vi "Run Command Gavin.vi"(2 "Line Index In":i32, 3 "Script":string) -> (0 "Line Index Out":i32, 1 "Done":bool)   [LabVIEW 2017, in "Apple script.lvlib"]
doc: "Looks at a line and runs the appropriate command. Add new commands to this vi."
uses:
  Apple script.lvlib
  Robot Global Data.vi
  <vilib>/addons/control/pid/pid.llb/PID.vi
  <vilib>/addons/control/pid/pid.llb/PID (DBL).vi
  Support Code/Angle Distance.vi
  Support Code/Pigeon Gyro.vi
  Support Code/Encoders.vi
  <vilib>/Rock Robotics/Network Tables/NT Write Value.vi
  <vilib>/Rock Robotics/Network Tables/NT Write Numeric Array.vi
  Parse Number.vi
  Timer.vi
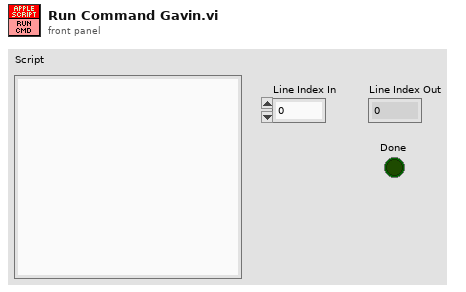
[diagram p1: front panel]
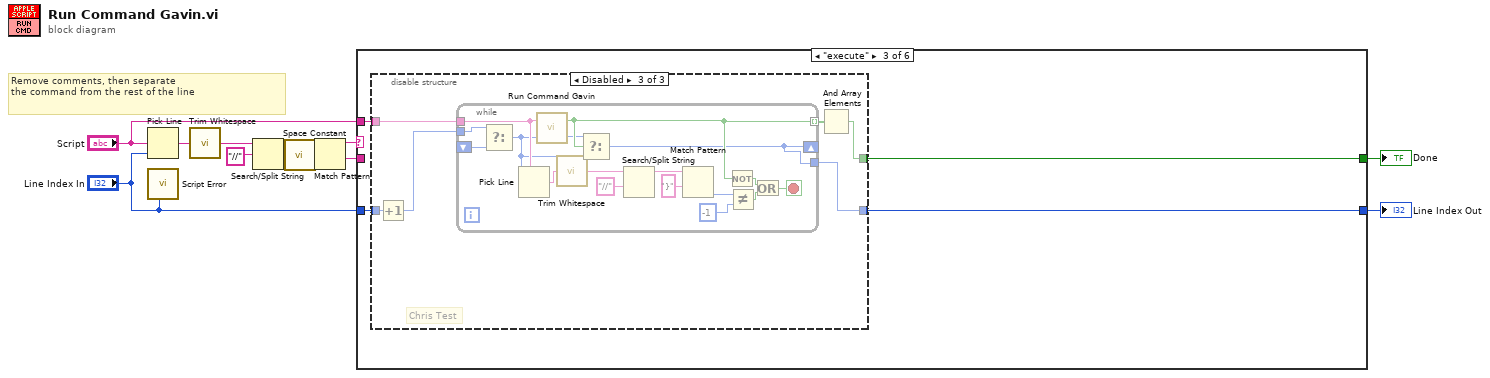
[diagram p0: block diagram]
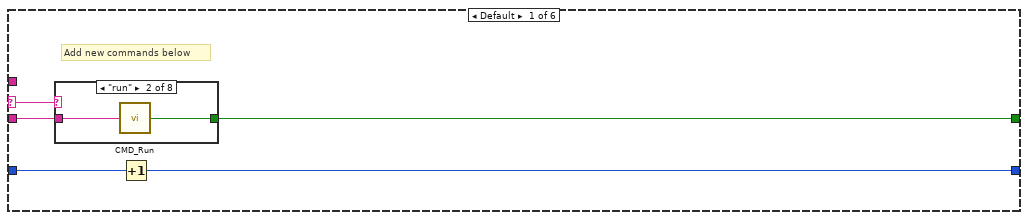
[diagram p2: hidden frame]
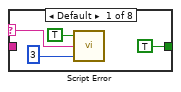
[diagram p3: hidden frame]
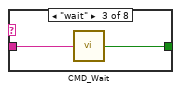
[diagram p4: hidden frame]
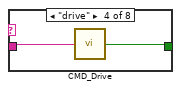
[diagram p5: hidden frame]
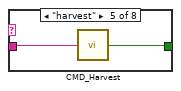
[diagram p6: hidden frame]
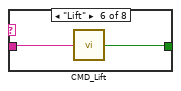
[diagram p7: hidden frame]
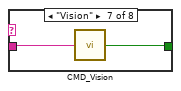
[diagram p8: hidden frame]
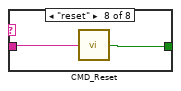
[diagram p9: hidden frame]
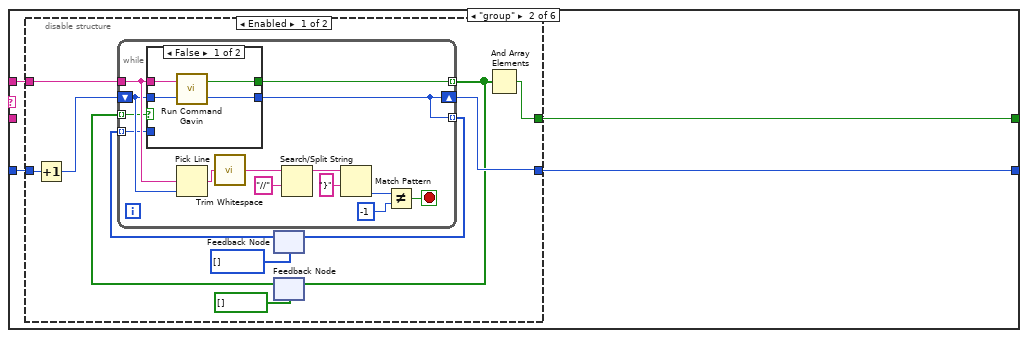
[diagram p10: hidden frame]
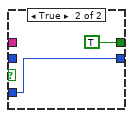
[diagram p11: hidden frame]
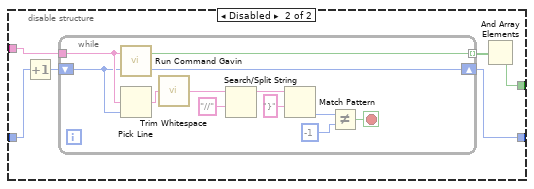
[diagram p12: hidden frame]
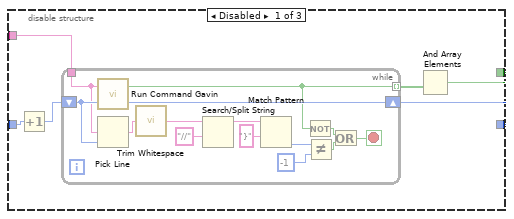
[diagram p13: hidden frame]
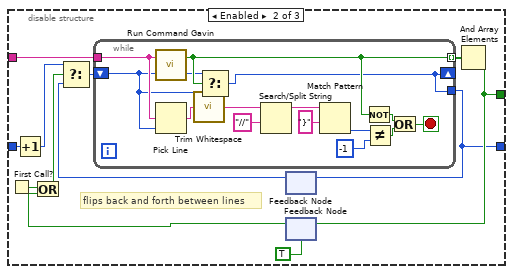
[diagram p14: hidden frame]
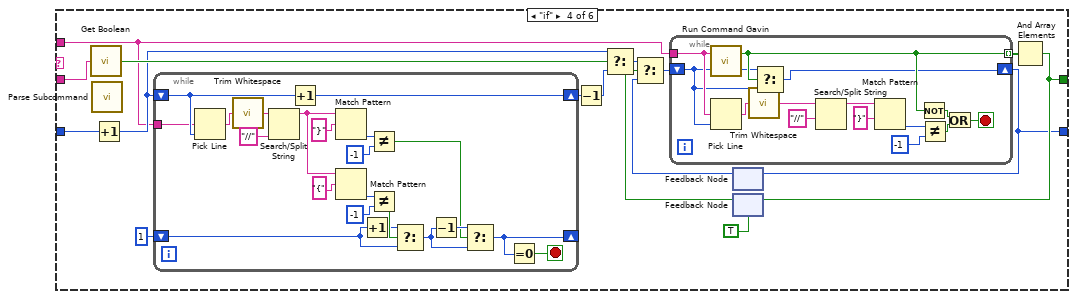
[diagram p15: hidden frame]
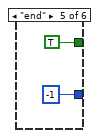
[diagram p16: hidden frame]
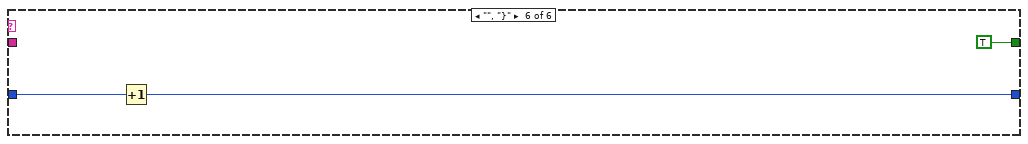
[diagram p17: hidden frame]
diagram:
  # "Remove comments, then separate\nthe command from the rest of the line"
  n1 = Pick Line(multi-line string="Script", line index="Line Index In") -> (output string=w8:string)  [unwired: 1 in]
  n2 = call "Script Error.vi"("Line Number"="Line Index In") -> ()  [unwired: 4 in, 1 out]
  n3 = call <vilib>:"Trim Whitespace.vi"("string"=w8) -> ("trimmed string"=w6:string)  [unwired: 1 in]
  n4 = Search/Split String(string=w6, search string/char (-)="//") -> (substring before match=w5:string)  [unwired: 1 in, 2 out]
  n5 = call <vilib>:"Space Constant.vi"() -> ("String"=w11:string)
  n6 = Match Pattern(string=w5, regular expression=w11) -> (before substring=w4:string, after substring=w3:string)  [unwired: 1 in, 2 out]
  n7 = case shown="\"execute\"" w4 {
    selector: w4 -> [w14 _ _ _ _ _]
    tunnel: "Script" -> [_ w38 w88 w164 _ _]
    tunnel: "Line Index In" -> [w16 w36 w89 w176 _ w217]
    tunnel: [w13 w35 w91 w177 TRUE ("Running") TRUE ("Running")] -> w2
    tunnel: [w15 w37 w90 w174 -1 ("Line Index Out") w216] -> w1
    tunnel: w3 -> [w12 _ _ w175 _ _]
    frame Default {
      # "Add new commands below"
      n8 = case shown="\"run\"" w14 {
        selector: w14 -> [w17 _ _ _ _ _ _ _]
        tunnel: [TRUE w21 w24 w25 w27 w29 w31 w33] -> w13
        tunnel: w12 -> [_ w22 w23 w26 w28 w30 w32 w34]
        frame Default {
          n9 = call "Script Error.vi"("Error?"=TRUE, "Error Details"=w17, "Error Code"=3) -> ()  [unwired: 2 in, 1 out]
        }
        frame "run" {
          n10 = call "CMD_Run.vi"("Line"=w22) -> ("Done"=w21:bool)
        }
        frame "wait" {
          n11 = call "CMD_Wait.vi"("Line"=w23) -> ("Done"=w24:bool)
        }
        frame "drive" {
          n12 = call "CMD_Drive.vi"("Line"=w26) -> ("Done"=w25:bool)
        }
        frame "harvest" {
          n13 = call "CMD_Harvest.vi"("Line"=w28) -> ("Done"=w27:bool)
        }
        frame "Lift" {
          n14 = call "CMD_Lift.vi"("Line"=w30) -> ("Done"=w29:bool)
        }
        frame "Vision" {
          n15 = call "CMD_Vision.vi"("Line"=w32) -> ("Done"=w31:bool)
        }
        frame "reset" {
          n16 = call "CMD_Reset.vi"("Line"=w34) -> ("Done"=w33:bool)
        }
      }
      n17 = Increment(x=w16) -> (x+1=w15:i32)
    }
    frame "group" {
      n18 = disable-structure shown="Enabled" {
        disable-tunnel: w38 -> [w47 w75]
        disable-tunnel: [w48 w72] -> w37
        disable-tunnel: w36 -> [w46 w74]
        disable-tunnel: [w49 w70] -> w35
        frame Enabled {
          n19 = Increment(x=w46) -> (x+1=w42:i32)
          n20 = feedback #1(i32[] []) -> (w41:i32[])
          n21 = feedback #2(bool[] []) -> (w44:bool[])
          n22 = while {
            tunnel: w47 -> [w63]
            tunnel: [w56] -> w45 mode=indexing
            shift-right: [w51] -> w48
            shift-left: w42 -> [w55]
            tunnel: w44 -> [w52] mode=indexing
            tunnel: [w51] -> w43 mode=indexing
            tunnel: w41 -> [w50] mode=indexing
            stop <- w53 stop-if-true
            n23 = case shown="False" w52 {
              tunnel: w63 -> [w67 _]
              tunnel: [w66 TRUE ("Done")] -> w56
              tunnel: w55 -> [w65 _]
              tunnel: [w64 w68] -> w51
              tunnel: w50 -> [_ w68]
              frame False {
                n24 = call "Run Command Gavin.vi"("Line Index In"=w65, "Script"=w67) -> ("Line Index Out"=w64:i32, "Done"=w66:bool)
              }
              frame True {
              }
            }
            n25 = Pick Line(multi-line string=w63, line index=w55) -> (output string=w58:string)  [unwired: 1 in]
            n26 = call <vilib>:"Trim Whitespace.vi"("string"=w58) -> ("trimmed string"=w59:string)  [unwired: 1 in]
            n27 = Search/Split String(string=w59, search string/char (-)="//") -> (substring before match=w54:string)  [unwired: 1 in, 2 out]
            n28 = Match Pattern(string=w54, regular expression="}" ("search string/char (-)")) -> (offset past match=w61:i32)  [unwired: 1 in, 3 out]
            n29 = Not Equal?(x=w61, y=-1) -> (x != y?=w53:bool)
          }
          n30 = feedback-in #1(w43) -> ()
          n31 = feedback-in #2(w45) -> ()
          n32 = And Array Elements(Boolean array=w45) -> (logical AND=w49:bool)
        }
        frame Disabled {
          n33 = Increment(x=w74) -> (x+1=w73:i32)
          n34 = while {
            tunnel: w75 -> [w87]
            tunnel: [w80] -> w71 mode=indexing
            shift-right: [w77] -> w72
            shift-left: w73 -> [w79]
            stop <- w78 stop-if-true
            n35 = call "Run Command Gavin.vi"("Line Index In"=w79, "Script"=w87) -> ("Line Index Out"=w77:i32, "Done"=w80:bool)
            n36 = Pick Line(multi-line string=w87, line index=w79) -> (output string=w82:string)  [unwired: 1 in]
            n37 = call <vilib>:"Trim Whitespace.vi"("string"=w82) -> ("trimmed string"=w83:string)  [unwired: 1 in]
            n38 = Search/Split String(string=w83, search string/char (-)="//") -> (substring before match=w76:string)  [unwired: 1 in, 2 out]
            n39 = Match Pattern(string=w76, regular expression="}" ("search string/char (-)")) -> (offset past match=w85:i32)  [unwired: 1 in, 3 out]
            n40 = Not Equal?(x=w85, y=-1) -> (x != y?=w78:bool)
          }
          n41 = And Array Elements(Boolean array=w71) -> (logical AND=w70:bool)
        }
      }
    }
    frame "execute" {
      n42 = disable-structure shown="Disabled" {
        disable-tunnel: [w94 w116 w141] -> w91
        disable-tunnel: [w95 w112 w139] -> w90
        disable-tunnel: w89 -> [w93 w123 w144]
        disable-tunnel: w88 -> [w96 w121 w142]
        frame Disabled {
          n43 = Increment(x=w93) -> (x+1=w92:i32)
          n44 = while {
            tunnel: w96 -> [w103]
            tunnel: [w99] -> w97 mode=indexing
            shift-right: [w111] -> w95
            shift-left: w92 -> [w104]
            stop <- w102 stop-if-true
            n45 = call "Run Command Gavin.vi"("Line Index In"=w104, "Script"=w103) -> ("Line Index Out"=w111:i32, "Done"=w99:bool)
            n46 = Pick Line(multi-line string=w103, line index=w104) -> (output string=w106:string)  [unwired: 1 in]
            n47 = call <vilib>:"Trim Whitespace.vi"("string"=w106) -> ("trimmed string"=w107:string)  [unwired: 1 in]
            n48 = Search/Split String(string=w107, search string/char (-)="//") -> (substring before match=w98:string)  [unwired: 1 in, 2 out]
            n49 = Match Pattern(string=w98, regular expression="}" ("search string/char (-)")) -> (offset past match=w109:i32)  [unwired: 1 in, 3 out]
            n50 = Not(x=w99) -> (.not. x?=w100:bool)
            n51 = Not Equal?(x=w109, y=-1) -> (x != y?=w101:bool)
            n52 = Or(x=w100, y=w101) -> (x .or. y?=w102:bool)
          }
          n53 = And Array Elements(Boolean array=w97) -> (logical AND=w94:bool)
        }
        frame Enabled {
          # "flips back and forth between lines"
          n54 = First Call?() -> (First Call?: T/F=w113:bool)
          n55 = Increment(x=w123) -> (x+1=w119:i32)
          n56 = feedback #3() -> (w118:i32)  [unwired: 1 in]
          n57 = feedback #4(TRUE) -> (w117:bool)
          n58 = Or(x=w113, y=w117) -> (x .or. y?=w114:bool)
          n59 = Select(t=w119, s=w114, f=w118) -> (s? t:f=w120:i32)
          n60 = while {
            tunnel: w121 -> [w138]
            tunnel: [w128] -> w122 mode=indexing
            shift-right: [w124] -> _
            shift-left: w120 -> [w126]
            tunnel: [w124] -> w112
            stop <- w137 stop-if-true
            n61 = call "Run Command Gavin.vi"("Line Index In"=w126, "Script"=w138) -> ("Line Index Out"=w127:i32, "Done"=w128:bool)
            n62 = Pick Line(multi-line string=w138, line index=w126) -> (output string=w132:string)  [unwired: 1 in]
            n63 = call <vilib>:"Trim Whitespace.vi"("string"=w132) -> ("trimmed string"=w133:string)  [unwired: 1 in]
            n64 = Select(t=w127, s=w128, f=w126) -> (s? t:f=w124:i32)
            n65 = Search/Split String(string=w133, search string/char (-)="//") -> (substring before match=w125:string)  [unwired: 1 in, 2 out]
            n66 = Match Pattern(string=w125, regular expression="}" ("search string/char (-)")) -> (offset past match=w135:i32)  [unwired: 1 in, 3 out]
            n67 = Not(x=w128) -> (.not. x?=w129:bool)
            n68 = Not Equal?(x=w135, y=-1) -> (x != y?=w130:bool)
            n69 = Or(x=w129, y=w130) -> (x .or. y?=w137:bool)
          }
          n70 = feedback-in #3(w112) -> ()
          n71 = And Array Elements(Boolean array=w122) -> (logical AND=w116:bool)
          n72 = feedback-in #4(w116) -> ()
        }
        frame Disabled {
          # "Chris Test"
          n73 = Increment(x=w144) -> (x+1=w140:i32)
          n74 = while {
            tunnel: w142 -> [w161]
            tunnel: [w151] -> w143 mode=indexing
            shift-right: [w145] -> _
            shift-left: _ -> [w146]
            tunnel: w140 -> [w148]
            tunnel: [w145] -> w139
            stop <- w160 stop-if-true
            n75 = Select(t=w148, f=w146) -> (s? t:f=w147:i32)  [unwired: 1 in]
            n76 = Pick Line(multi-line string=w161, line index=w147) -> (output string=w155:string)  [unwired: 1 in]
            n77 = call "Run Command Gavin.vi"("Line Index In"=w147, "Script"=w161) -> ("Line Index Out"=w150:i32, "Done"=w151:bool)
            n78 = call <vilib>:"Trim Whitespace.vi"("string"=w155) -> ("trimmed string"=w156:string)  [unwired: 1 in]
            n79 = Select(t=w150, s=w151, f=w147) -> (s? t:f=w145:i32)
            n80 = Search/Split String(string=w156, search string/char (-)="//") -> (substring before match=w149:string)  [unwired: 1 in, 2 out]
            n81 = Match Pattern(string=w149, regular expression="}" ("search string/char (-)")) -> (offset past match=w158:i32)  [unwired: 1 in, 3 out]
            n82 = Not(x=w151) -> (.not. x?=w152:bool)
            n83 = Not Equal?(x=w158, y=-1) -> (x != y?=w153:bool)
            n84 = Or(x=w152, y=w153) -> (x .or. y?=w160:bool)
          }
          n85 = And Array Elements(Boolean array=w143) -> (logical AND=w141:bool)
        }
      }
    }
    frame "if" {
      n86 = call "Get Boolean.vi"("Name"=w175) -> ("Value"=w168:bool)
      n87 = call "Parse Subcommand.vi"() -> ()  [unwired: 9 in, 7 out]
      n88 = Increment(x=w176) -> (x+1=w166:i32)
      n89 = while {
        shift-right: [w191] -> w165
        shift-left: w166 -> [w193]
        shift-right: [w179] -> _
        shift-left: 1 -> [w184]
        tunnel: w164 -> [w178]
        stop <- w180 stop-if-true
        n90 = Pick Line(multi-line string=w178, line index=w193) -> (output string=w195:string)  [unwired: 1 in]
        n91 = call <vilib>:"Trim Whitespace.vi"("string"=w195) -> ("trimmed string"=w196:string)  [unwired: 1 in]
        n92 = Search/Split String(string=w196, search string/char (-)="//") -> (substring before match=w187:string)  [unwired: 1 in, 2 out]
        n93 = Increment(x=w193) -> (x+1=w191:i32)
        n94 = Match Pattern(string=w187, regular expression="}" ("search string/char (-)")) -> (offset past match=w198:i32)  [unwired: 1 in, 3 out]
        n95 = Match Pattern(string=w187, regular expression="{" ("search string/char (-)")) -> (offset past match=w188:i32)  [unwired: 1 in, 3 out]
        n96 = Increment(x=w184) -> (x+1=w185:i32)
        n97 = Not Equal?(x=w198, y=-1) -> (x != y?=w181:bool)
        n98 = Not Equal?(x=w188, y=-1) -> (x != y?=w186:bool)
        n99 = Select(t=w185, s=w186, f=w184) -> (s? t:f=w182:i32)
        n100 = Decrement(x=w182) -> (x-1=w183:i32)
        n101 = Select(t=w183, s=w181, f=w182) -> (s? t:f=w179:i32)
        n102 = Equal To 0?(x=w179) -> (x = 0?=w180:bool)
      }
      n103 = Decrement(x=w165) -> (x-1=w162:i32)
      n104 = Select(t=w166, s=w168, f=w162) -> (s? t:f=w169:i32)
      n105 = feedback #5() -> (w170:i32)  [unwired: 1 in]
      n106 = feedback #6(TRUE) -> (w173:bool)
      n107 = Select(t=w169, s=w173, f=w170) -> (s? t:f=w172:i32)
      n108 = while {
        tunnel: w164 -> [w213]
        tunnel: [w203] -> w171 mode=indexing
        shift-right: [w200] -> w174
        shift-left: w172 -> [w201]
        stop <- w212 stop-if-true
        n109 = call "Run Command Gavin.vi"("Line Index In"=w201, "Script"=w213) -> ("Line Index Out"=w202:i32, "Done"=w203:bool)
        n110 = Pick Line(multi-line string=w213, line index=w201) -> (output string=w207:string)  [unwired: 1 in]
        n111 = call <vilib>:"Trim Whitespace.vi"("string"=w207) -> ("trimmed string"=w208:string)  [unwired: 1 in]
        n112 = Select(t=w202, s=w203, f=w201) -> (s? t:f=w200:i32)
        n113 = Search/Split String(string=w208, search string/char (-)="//") -> (substring before match=w199:string)  [unwired: 1 in, 2 out]
        n114 = Match Pattern(string=w199, regular expression="}" ("search string/char (-)")) -> (offset past match=w210:i32)  [unwired: 1 in, 3 out]
        n115 = Not(x=w203) -> (.not. x?=w204:bool)
        n116 = Not Equal?(x=w210, y=-1) -> (x != y?=w205:bool)
        n117 = Or(x=w204, y=w205) -> (x .or. y?=w212:bool)
      }
      n118 = feedback-in #5(w174) -> ()
      n119 = And Array Elements(Boolean array=w171) -> (logical AND=w177:bool)
      n120 = feedback-in #6(w177) -> ()
    }
    frame "end" {
    }
    frame "", "}" {
      n121 = Increment(x=w217) -> (x+1=w216:i32)
    }
  }
  "Line Index Out" <- w1
  "Done" <- w2
